vi "Read Coils.vi"(8 "error in (no error)":errorcluster, 9 "number of coils":u16, 10 "address":u16, 11 "MODBUS in":refnum<class "PL Modbus Client.lvclass">) -> (0 "error out":errorcluster, 2 "values":bool[](array[boolean]), 3 "MODBUS out":refnum<class "PL Modbus Client.lvclass">)   [LabVIEW 2015, in "PL Modbus Client.lvclass"]
doc: "Reads a specified <B>number of coils</B> starting at specified <B>address</B> (Modbus function code: <B>1</B>)."
uses:
  PL Modbus Client.lvclass
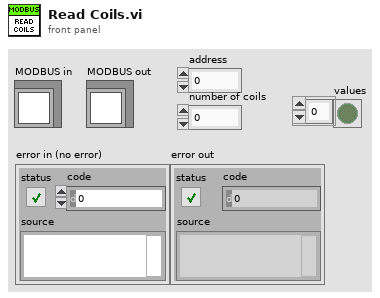
[diagram p1: front panel]
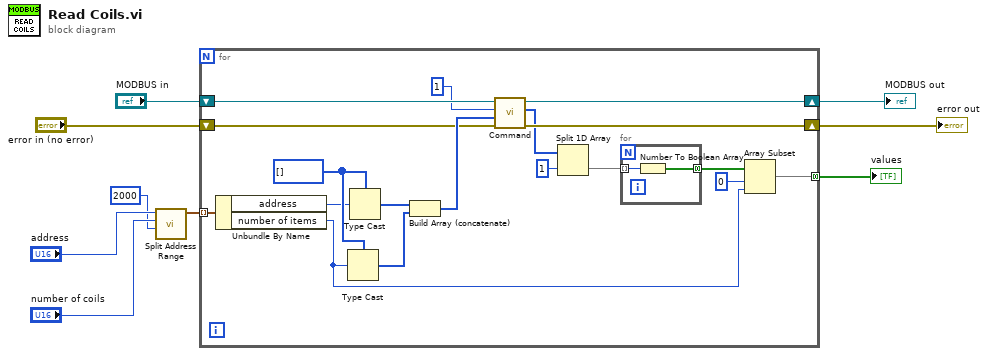
[diagram p0: block diagram]
diagram:
  n1 = call "Split Address Range.vi"("max number of items"=u16 2000, "number of items"="number of coils", "address"="address") -> ("addresses and numbers of items"=w3:cluster{"address":u16, "number of items":u16}[])  [unwired: 8 in]
  n2 = for {
    tunnel: [w13] -> w7 mode=concatenating
    shift-right: [w21] -> w8
    shift-left: "MODBUS in" -> [w27]
    shift-right: [w19] -> w1
    shift-left: "error in (no error)" -> [w20]
    tunnel: w3 -> [w12] mode=indexing
    w26 = u8[] []
    n3 = Unbundle By Name(w12) -> ("address"=w11:u16, "number of items"=w10:u16)
    n4 = Type Cast(type=w26, x=w10) -> (*(type *) &x=w24:u8[])
    n5 = Type Cast(type=w26, x=w11) -> (*(type *) &x=w25:u8[])
    n6 = Build Array (concatenate)(w25, w24) -> (w23:u8[])
    n7 = call-dynamic "Command.vi"("error in (no error)"=w20, "data in"=w23, "function code"=u8 1 ("function"), "MODBUS in"=w27) -> ("error out"=w19:errorcluster, "data out"=w18:u8[], "MODBUS out"=w21:refnum<class "PL Modbus Client.lvclass">)  [unwired: 5 in]
    n8 = Split 1D Array(array=w18, index=1) -> (second subarray=w15:u8[])  [unwired: 1 out]
    n9 = for {
      tunnel: [w28] -> _ mode=indexing
      tunnel: [w29] -> w14 mode=concatenating
      tunnel: w15 -> [w28] mode=indexing
      n10 = Number To Boolean Array(number=w28) -> (Boolean array=w29:bool[])
    }
    n11 = Array Subset(array=w14, index=0, length=w10) -> (w13:bool[])
  }
  "MODBUS out" <- w8
  "values" <- w7
  "error out" <- w1
